vi "GET.issues.vi"(8 "error in (no error)":errorcluster, 11 "issue_class in":refnum<class "issue_class.lvclass">) -> (0 "error out":errorcluster, 3 "issue_class out":refnum<class "issue_class.lvclass">)   [LabVIEW 2024, in "issue_class.lvclass"]
uses:
  issue_class.lvclass
  issue_class.lvclass/issue_class.ctl
panel:
  out "current url":string
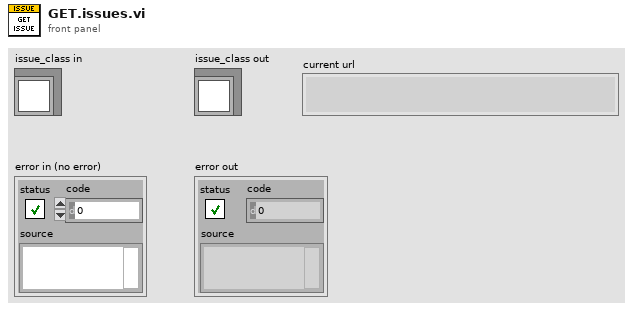
[diagram p1: front panel]
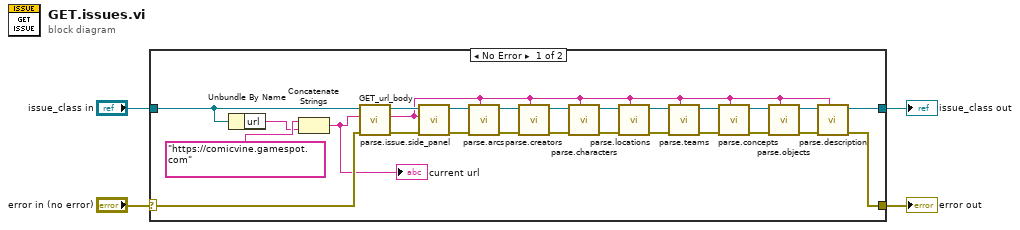
[diagram p0: block diagram]
diagram:
  n1 = case shown="No Error" "error in (no error)" {
    selector: "error in (no error)" -> [w29 w32]
    tunnel: [w6 w32] -> w3
    tunnel: [w8 w31] -> w1
    tunnel: "issue_class in" -> [w30 w31]
    frame No Error {
      n2 = Unbundle By Name(w30) -> ("url"=w10:string)
      n3 = Concatenate Strings("https://comicvine.gamespot.com", w10) -> (w12:string)
      "current url" <- w12
      n4 = call-dynamic "GET_url_body.vi"("error in (no error)"=w29, "url"=w12, "comic_class in"=w30) -> ("error out"=w27:errorcluster, "body"=w5:string, "comic_class out"=w28:refnum<class "issue_class.lvclass">)  [unwired: 6 in]
      n5 = call "parse.issue.side_panel.vi"("error in (no error)"=w27, "body"=w5, "issue_class in"=w28) -> ("error out"=w19:errorcluster, "issue_class out"=w26:refnum<class "issue_class.lvclass">)  [unwired: 7 in]
      n6 = call "parse.arcs.vi"("body"=w5, "error in (no error)"=w19, "issue_class in"=w26) -> ("error out"=w18:errorcluster, "issue_class out"=w25:refnum<class "issue_class.lvclass">)  [unwired: 7 in]
      n7 = call "parse.creators.vi"("body"=w5, "error in (no error)"=w18, "issue_class in"=w25) -> ("error out"=w17:errorcluster, "issue_class out"=w24:refnum<class "issue_class.lvclass">)  [unwired: 7 in]
      n8 = call "parse.characters.vi"("body"=w5, "error in (no error)"=w17, "issue_class in"=w24) -> ("error out"=w16:errorcluster, "issue_class out"=w23:refnum<class "issue_class.lvclass">)  [unwired: 7 in]
      n9 = call "parse.locations.vi"("body"=w5, "error in (no error)"=w16, "issue_class in"=w23) -> ("error out"=w15:errorcluster, "issue_class out"=w22:refnum<class "issue_class.lvclass">)  [unwired: 7 in]
      n10 = call "parse.teams.vi"("body"=w5, "error in (no error)"=w15, "issue_class in"=w22) -> ("error out"=w14:errorcluster, "issue_class out"=w21:refnum<class "issue_class.lvclass">)  [unwired: 7 in]
      n11 = call "parse.concepts.vi"("body"=w5, "error in (no error)"=w14, "issue_class in"=w21) -> ("error out"=w13:errorcluster, "issue_class out"=w20:refnum<class "issue_class.lvclass">)  [unwired: 7 in]
      n12 = call "parse.objects.vi"("body"=w5, "error in (no error)"=w13, "issue_class in"=w20) -> ("error out"=w7:errorcluster, "issue_class out"=w9:refnum<class "issue_class.lvclass">)  [unwired: 7 in]
      n13 = call "parse.description.vi"("body"=w5, "error in (no error)"=w7, "issue_class in"=w9) -> ("error out"=w6:errorcluster, "issue_class out"=w8:refnum<class "issue_class.lvclass">)  [unwired: 7 in]
    }
    frame Error {
    }
  }
  "error out" <- w3
  "issue_class out" <- w1
